vi "Initialize.vi"(8 "error in":errorcluster, 10 "shared resources":refnum<class "Shared Resources.lvclass">, 11 "tx execution unit":refnum<class "Tx Execution Unit.lvclass">) -> (0 "error out":errorcluster, 3 "tx execution unit out":refnum<class "Tx Execution Unit.lvclass">)   [LabVIEW 2020, in "AIM MIL-STD-1553 Engine.lvlib" / "Implementation.lvlib" / "Tx Execution Unit.lvclass"]
uses:
  Tx Execution Unit.lvclass
  Execution Unit/Execution Unit.lvclass
  Interfaces/Shared Resources/Shared Resources.lvclass
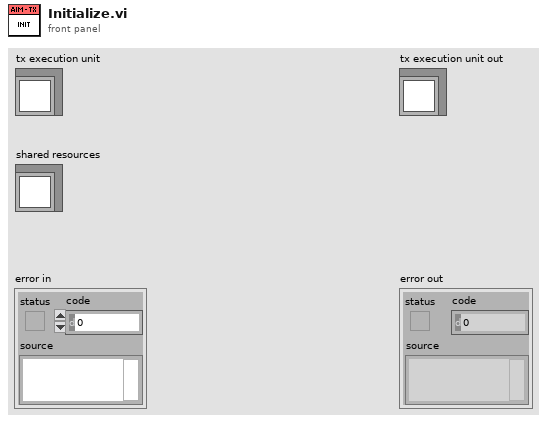
[diagram p1: front panel]
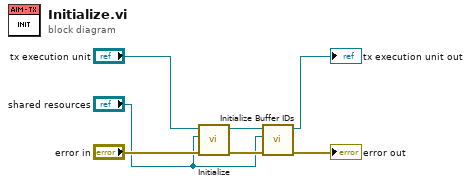
[diagram p0: block diagram]
diagram:
  n1 = call-parent "Initialize.vi"("error in"="error in", "shared resources"="shared resources", "Execution Unit Implementation in"="tx execution unit") -> ("error out"=w4:errorcluster, "Execution Unit Implementation out"=w6:refnum<class "Tx Execution Unit.lvclass">)  [unwired: 7 in]
  n2 = call "Initialize Buffer IDs.vi"("error in (no error)"=w4, "shared resources"="shared resources", "Tx Execution Unit in"=w6) -> ("error out"=→"error out":errorcluster, "Tx Execution Unit out"=→"tx execution unit out":refnum<class "Tx Execution Unit.lvclass">)  [unwired: 7 in]
